vi "HFRR ADV v036.vi"() -> ()   [LabVIEW 2025] (continued)
                n905 = Match Pattern(string=w1143, regular expression=" \"width_px\":") -> (after substring=w1141:string)  [unwired: 1 in, 3 out]
                n906 = Match Pattern(string=w1141, regular expression="\"height_px\":") -> (before substring=w1139:string, after substring=w1138:string)  [unwired: 1 in, 2 out]
                n907 = Fract/Exp String To Number(string=w1139, default (0 dbl)=w1137) -> (number=w1136:dbl)  [unwired: 2 in, 1 out]
                n908 = Fract/Exp String To Number(string=w1138, default (0 dbl)=w1137) -> (number=w1135:dbl)  [unwired: 2 in, 1 out]
                n909 = Multiply(x=w1136, y=w1134) -> (x*y=w1133:dbl)
                n910 = Multiply(x=w1135, y=w1134) -> (x*y=w1132:dbl)
                n911 = Multiply(x=w1133, y=w1131) -> (x*y=w1117:dbl)
                n912 = Multiply(x=w1132, y=w1131) -> (x*y=w1115:dbl)
                n913 = Add(x=w1117, y=w1115) -> (x+y=w1129:dbl)
                n914 = property on="Major Axis" class="DigNum (strict)"("Caption.Text"="Major Axis") -> ()  [unwired: 2 in, 2 out]
                n915 = property on="Minor Axis" class="DigNum (strict)"("Caption.Text"="Minor Axis") -> ()  [unwired: 2 in, 2 out]
                n916 = property on="Average" class="DigNum (strict)"("Caption.Text"="Average") -> ()  [unwired: 2 in, 2 out]
                n917 = Divide(x=w1129, y=2.0) -> (x/y=w1113:dbl)
                n918 = Bundle By Name(cluster=w1130, "major"=w1117, "minor"=w1115, "average"=w1113) -> (w1127:cluster{"major":dbl, "minor":dbl, "average":dbl})
                n919 = Number To Fractional String(number=w1115, precision (6)=i16 1) -> (F-format string=w1122:string)  [unwired: 2 in]
                n920 = Number To Fractional String(number=w1113, precision (6)=i16 1) -> (F-format string=w1123:string)  [unwired: 2 in]
                n921 = Number To Fractional String(number=w1117, precision (6)=i16 1) -> (F-format string=w1121:string)  [unwired: 2 in]
                n922 = Fract/Exp String To Number(string=w1122) -> (number=w1114:dbl)  [unwired: 3 in, 1 out]
                n923 = Fract/Exp String To Number(string=w1123) -> (number=w1112:dbl)  [unwired: 3 in, 1 out]
                n924 = Fract/Exp String To Number(string=w1121) -> (number=w1116:dbl)  [unwired: 3 in, 1 out]
                n925 = local write "Major Axis"(w1116) -> ()
                n926 = local write "Average"(w1112) -> ()
                n927 = local write "Minor Axis"(w1114) -> ()
              }
            }
            n928 = case shown="\"Measrument\", Default" w1026 {
              tunnel: w1029 -> [w1056 _]
              tunnel: w1028 -> [w1055 _]
              tunnel: [w1052 w1081] -> w1027
              tunnel: w1025 -> [w1054 w1081]
              tunnel: w1024 -> [w1053 _]
              tunnel: w1021 -> [w1051 _]
              frame "Measrument", Default {
                n929 = stacked-sequence {
                  tunnel: w1056 -> [w1074 _]
                  tunnel: w1055 -> [w1072 _]
                  tunnel: w1054 -> [w1070 _]
                  tunnel: w1053 -> [w1069 _]
                  tunnel: [w1064 _] -> w1052
                  tunnel: w1051 -> [w1057 _]
                  frame #0 {
                    n930 = call "IMAGE ANALYSIS.vi"("Enum"=POST_ANALYSIS_ENUM."SAVE IMAGE", "error in"=w1070, "IMAGE FILE PATH"=w1069) -> ("error out"=w1068:errorcluster)  [unwired: 7 in, 1 out]
                    n931 = call "Stall Data Flow.vim"("value in"=w1068, "milliseconds to wait"=u32 1000) -> ("value out"=w1059:errorcluster)  [unwired: 1 out]
                    n932 = local read "Test File List :"() -> (w1076:string)
                    n933 = call "IMAGE ANALYSIS.vi"("Enum"=POST_ANALYSIS_ENUM."MINIMIZE UI", "error in"=w1059) -> ("error out"=w1066:errorcluster)  [unwired: 8 in, 1 out]
                    n934 = Bundle By Name(cluster=T27 {"File Name"="", "Test Method"="", "Operator"="", "Fuel Description"="", "Date and time"=""} ("Main Ref"), "Test Method"=w1057, "File Name"=w1076) -> (w1077:T27)
                    n935 = call "Stall Data Flow.vim"("value in"=w1066, "milliseconds to wait"=u32 1500) -> ("value out"=w1061:errorcluster)  [unwired: 1 out]
                    n936 = call "duf file read.vi"("error in (no error)"=w1061, "Main Ref"=w1077) -> ("error out"=w1075:errorcluster, "Main Ref 2"=w1073:T27)  [unwired: 8 in]
                    n937 = call "DETECTION REPORT for manual.vi"("error in (no error)"=w1075, "return value 3"=w1072, "Image File Path"=w1074, "Main Ref"=w1073) -> ("error out"=w1071:errorcluster)  [unwired: 7 in]
                    n938 = call <vilib>:"Clear Errors.vi"("error in (no error)"=w1071) -> ("error out"=w1062:errorcluster)  [unwired: 5 in, 1 out]
                    n939 = call "IMAGE ANALYSIS.vi"("Enum"=POST_ANALYSIS_ENUM."MINIMIZE UI", "error in"=w1062) -> ("error out"=w1064:errorcluster)  [unwired: 8 in, 1 out]
                  }
                  frame #1 {
                    n940 = local write "Main Tab"(T2."HOME" ("Main Tab")) -> ()
                    n941 = local write "Main Dashboard Buttons"(T1."Home" ("Main Dashboard Buttons")) -> ()
                  }
                }
              }
              frame "Calibrate" {
              }
            }
          }
          frame #2 {
            n942 = Not(x=w1146) -> (.not. x?=w1145:bool)
            n943 = local write "Confirm Measrurement"(w1145) -> ()
            n944 = local read "Calibration Tab"() -> (w1144:enum32{"Measrument", "Calibrate"})
            n945 = case shown="\"Measrument\", Default" w1144 {
              frame "Measrument", Default {
                (unwired) T21."HOME" ("Main Tab")
                n946 = local write "Main Tab"(T2."HOME" ("Main Tab")) -> ()
              }
              frame "Calibrate" {
              }
            }
          }
        }
      }
    }
    n947 = local read "Humidity"() -> (w889:bool)
    n948 = local read "Save Change"() -> (w894:bool)
    n949 = local read "Calibrate"() -> (w895:bool)
    n950 = local read "Auto Start Test"() -> (w890:bool)
    n951 = case shown="True" w895 {
      selector: w895 -> [_ w1002]
      frame False {
      }
      frame True {
        n952 = Not(x=w1002) -> (.not. x?=w1001:bool)
        n953 = local write "Calibrate"(w1001) -> ()
        n954 = local write "Calibration Tab"(enum32{"Measrument", "Calibrate"}."Calibrate" ("Calibration Tab")) -> ()
      }
    }
    n955 = case shown="True" w894 {
      selector: w894 -> [_ w946]
      frame False {
      }
      frame True {
        n956 = stacked-sequence {
          tunnel: w946 -> [_ _ _ _ w1000]
          frame #0 {
            n957 = call "IMAGE ANALYSIS.vi"("Enum"=POST_ANALYSIS_ENUM."HIDE UI") -> ()  [unwired: 9 in, 2 out]
          }
          frame #1 {
            n958 = local read "100x gain"() -> (w948:dbl)
            n959 = local read "10x Gain"() -> (w949:dbl)
            n960 = local read "5x Gain"() -> (w950:dbl)
            n961 = Number To Fractional String(number=w949, width (-)=i16 4, precision (6)=i16 7) -> (F-format string=w971:string)  [unwired: 1 in]
            n962 = Number To Fractional String(number=0.0, width (-)=i16 4, precision (6)=i16 7) -> (F-format string=w966:string)  [unwired: 1 in]
            n963 = Number To Fractional String(number=w948, width (-)=i16 4, precision (6)=i16 7) -> (F-format string=w954:string)  [unwired: 1 in]
            n964 = Number To Fractional String(number=w950, width (-)=i16 10 ("precision (6)"), precision (6)=i16 7) -> (F-format string=w980:string)  [unwired: 1 in]
            n965 = Concatenate Strings("[CH1]" ("string"), w980, " - 5x Gain" ("string"), "\r") -> (w970:string)
            n966 = Concatenate Strings("[CH2]" ("string"), w971, " - 10x Gain" ("string"), "\r") -> (w969:string)
            n967 = Concatenate Strings("[CH3]" ("string"), w966, " - 20x Gain" ("string"), "\r") -> (w960:string)
            n968 = Concatenate Strings("[CH4]" ("string"), w954, " - 100x Gain" ("string"), "\r") -> (w953:string)
            n969 = String To Path(string="C:\\LAB-IQ\\Image Calibrate v01.dcf") -> (path=w983:path)
            n970 = Concatenate Strings(w970, w969, w960, w953) -> (w968:string)
            n971 = call <vilib>:"Write Characters To File.vi"("append to file? (new file:F)"=FALSE, "character string"=w968, "file path (dialog if empty)"=w983) -> ()  [unwired: 2 in, 1 out]
          }
          frame #2 {
            n972 = String To Path(string="C:\\LAB-IQ\\Image Calibrate v01.dcf") -> (path=w986:path)
            n973 = Open/Create/Replace File ("Open File")(file path (use dialog)=w986) -> (refnum out=w987:refnum<file>)  [unwired: 5 in, 2 out]
            n974 = for {
              N: 4 -> [_]
              tunnel: w987 -> [w993]
              i -> [w989]
              n975 = Read from Text File ("Read File")(file (use dialog)=w993) -> (text=w994:string)  [unwired: 3 in, 3 out]
              n976 = String Subset(string=w994, offset (0)=6, length (rest)=10 ("length (rest)")) -> (substring=w990:string)
              n977 = Fract/Exp String To Number(string=w990) -> (number=w988:dbl)  [unwired: 3 in, 1 out]
              n978 = case shown="3" w989 {
                tunnel: w988 -> [w995 w996 _ w997 _]
                frame 0 {
                  n979 = local write "5x Gain"(w995) -> ()
                }
                frame 1 {
                  n980 = local write "10x Gain"(w996) -> ()
                }
                frame 2 {
                }
                frame 3 {
                  n981 = local write "100x gain"(w997) -> ()
                }
                frame 4, Default {
                }
              }
            }
          }
          frame #3 {
            n982 = call "IMAGE ANALYSIS.vi"("Enum"=POST_ANALYSIS_ENUM."SHOW UI") -> ()  [unwired: 9 in, 2 out]
          }
          frame #4 {
            n983 = Not(x=w1000) -> (.not. x?=w999:bool)
            n984 = local write "Save Change"(w999) -> ()
          }
        }
      }
    }
    n985 = case shown="False" w890 {
      tunnel: w889 -> [w916 _]
      frame False {
        n986 = case shown="True" w916 {
          frame False {
          }
          frame True {
            n987 = local read "Set Humidity:"() -> (w920:dbl)
            n988 = local read "Set Humidity:"() -> (w923:dbl)
            n989 = local read "Humidity ( %RH )"() -> (w924:dbl)
            n990 = Subtract(x=w920, y=2.0) -> (x-y=w918:dbl)
            n991 = Add(x=w923, y=2.0) -> (x+y=w919:dbl)
            n992 = In Range and Coerce(upper limit=w919, x=w924, lower limit=w918) -> (In Range?=w917:bool)  [unwired: 1 out]
            n993 = case shown="True" w917 {
              frame False {
              }
              frame True {
                n994 = case shown="True" "Manual Humididty Reached" {
                  selector: "Manual Humididty Reached" -> [_ w927]
                  frame False {
                  }
                  frame True {
                    n995 = Not(x=w927) -> (.not. x?=w926:bool)
                    n996 = local write "Manual Humididty Reached"(w926) -> ()
                    n997 = local read "EVENT LOG"() -> (w929:string)
                    n998 = call "Event Log.vi"("Content"="Target Humidity reached", "EVENT LOG"=w929) -> ("EVENT LOG"=w928:string)  [unwired: 8 in, 1 out]
                    n999 = local write "EVENT LOG"(w928) -> ()
                  }
                }
              }
            }
          }
        }
      }
      frame True {
        n1000 = local write "Manual Humididty Reached"(TRUE ("Manual Humididty Reached")) -> ()
      }
    }
    n1001 = local read "Cap Live Image"() -> (w910:bool)
    n1002 = local read "SCAR MEASURMENT"() -> (w913:enum32{"Auto Scar", "Manual Scar"})
    n1003 = Wait (ms)(milliseconds to wait=u32 250) -> ()  [unwired: 1 out]
    n1004 = Equal?(x=w913, y=enum32{"Auto Scar", "Manual Scar"}."Manual Scar" ("SCAR MEASURMENT")) -> (x = y?=w911:bool)
    n1005 = And(x=w911, y=w910) -> (x .and. y?=w909:bool)
    n1006 = case shown="True" w909 {
      selector: w909 -> [_ w1225]
      frame False {
      }
      frame True {
        n1007 = stacked-sequence {
          tunnel: [_ _ _ w1240 _] -> _
          tunnel: w1225 -> [_ _ _ _ w1247]
          frame #0 {
            w1226 = 0.0
            n1008 = local write "Major Axis"(w1226) -> ()
            n1009 = local write "Minor Axis"(w1226) -> ()
            n1010 = local write "Average"(w1226) -> ()
          }
          frame #1 {
            n1011 = call "CAMERA LIVE FEED FGV.vi"("Enum - Menu"=CAMERA_LIVE_FEED_ENUM."CAMERA MINIMIZE") -> ()  [unwired: 9 in, 2 out]
          }
          frame #2 {
            n1012 = local read "FILE 3"() -> (w1234:string)
            n1013 = call <vilib>:"Trim Whitespace.vi"("string"="C:\\LAB-IQ\\images\\") -> ("trimmed string"=w1236:string)  [unwired: 1 in]
            n1014 = String To Path(string=w1236) -> (path=w1235:path)
            n1015 = Concatenate Strings(w1234, ".png" ("string")) -> (w1233:string)
            n1016 = Build Path(base path=w1235, name or relative path=w1233) -> (appended path=w1231:path)
            n1017 = Path To String(path=w1231) -> (string=w1230:string)
            n1018 = call "CAMERA LIVE FEED FGV.vi"("Enum - Menu"=CAMERA_LIVE_FEED_ENUM."CAMERA SAVE", "Image Path"=w1230) -> ("error out"=w1228:errorcluster)  [unwired: 8 in, 1 out]
            n1019 = case shown="No Error" w1228 {
              frame No Error {
                n1020 = One Button Dialog(message="Image saved successfully") -> ()  [unwired: 1 in, 1 out]
              }
              frame Error {
              }
            }
          }
          frame #3 {
            n1021 = call "LIST FILE NAMES.vi"() -> ("error out"=w1242:errorcluster, "filenames"=w1239:string[])  [unwired: 10 in]
            n1022 = call "IMAGE ANALYSIS.vi"("Enum"=POST_ANALYSIS_ENUM."SHOW UI", "error in"=w1242) -> ("error out"=w1240:errorcluster)  [unwired: 8 in, 1 out]
            n1023 = property on="Test File List :" class="CmbBox"("Strings[]"=w1239) -> ()  [unwired: 2 in, 2 out]
          }
          frame #4 {
            (unwired) T26."Report" ("Main Dashboard Buttons")
            (unwired) T28."Report" ("Main Dashboard Buttons")
            n1024 = Not(x=w1247) -> (.not. x?=w1246:bool)
            n1025 = local write "Zoom Factore"(0.0 ("Zoom Factore")) -> ()
            n1026 = local write "Cap Live Image"(w1246) -> ()
            n1027 = local write "Main Tab"(T2."Adv Scar Report" ("Main Tab")) -> ()
            n1028 = property on="Cap Live Image" class="Bool (strict)"("BoolText.Text"="Capture Image" ("Boolean Text.Text")) -> ()  [unwired: 2 in, 2 out]
            n1029 = local write "Main Dashboard Buttons"(T1."Report" ("Main Dashboard Buttons")) -> ()
          }
        }
      }
    }
    n1030 = local read "change Gain"() -> (w893:bool)
    n1031 = local read "Back Square"() -> (w892:bool)
    n1032 = case shown="True" w893 {
      selector: w893 -> [_ w937]
      frame False {
      }
      frame True {
        n1033 = stacked-sequence {
          tunnel: w937 -> [_ w945]
          frame #0 {
            n1034 = local read "Actual (µm)"() -> (w941:dbl)
            n1035 = local read "Pixel Value"() -> (w940:dbl)
            n1036 = local read "Magnification :"() -> (w939:string)
            n1037 = Divide(x=w941, y=w940) -> (x/y=w938:dbl)
            n1038 = case shown="\"10x\"" w939 {
              tunnel: w938 -> [w942 w943]
              frame "10x" {
                n1039 = local write "10x Gain"(w942) -> ()
              }
              frame "5x", Default {
                n1040 = local write "5x Gain"(w943) -> ()
              }
            }
          }
          frame #1 {
            n1041 = Not(x=w945) -> (.not. x?=w944:bool)
            n1042 = local write "change Gain"(w944) -> ()
          }
        }
      }
    }
    n1043 = case shown="True" w892 {
      selector: w892 -> [_ w935]
      frame False {
      }
      frame True {
        n1044 = Not(x=w935) -> (.not. x?=w934:bool)
        n1045 = local write "Back Square"(w934) -> ()
        n1046 = local write "Calibration Tab"(enum32{"Measrument", "Calibrate"}."Measrument" ("Calibration Tab")) -> ()
      }
    }
    n1047 = local read "Rectangle Tool"() -> (w904:bool)
    n1048 = local read "Clear ROI Tool"() -> (w903:bool)
    n1049 = local read "Open Image"() -> (w908:bool)
    n1050 = local read "line tool"() -> (w905:bool)
    n1051 = local read "OUT"() -> (w906:bool)
    n1052 = local read "In"() -> (w907:bool)
    n1053 = case shown="True" w908 {
      selector: w908 -> [_ w1213]
      tunnel: [w1209 w1215] -> _
      tunnel: w898 -> [w1209 w1214]
      frame False {
      }
      frame True {
        n1054 = Not(x=w1213) -> (.not. x?=w1212:bool)
        n1055 = local write "Open Image"(w1212) -> ()
        n1056 = call "IMAGE ANALYSIS.vi"("Enum"=POST_ANALYSIS_ENUM."HIDE UI", "error in"=w1214) -> ("error out"=w1222:errorcluster)  [unwired: 8 in, 1 out]
        n1057 = call "File Dialog"("start path"=path "C:/LAB-IQ/images", "error in"=w1222) -> ("selected path"=w1211:path, "error out"=w1220:errorcluster)  [unwired: 10 in, 2 out]
        "Image path  2" <- w1211
        n1058 = call <vilib>:"Clear Errors.vi"("error in (no error)"=w1220) -> ("error out"=w1219:errorcluster)  [unwired: 5 in, 1 out]
        n1059 = call "IMAGE ANALYSIS.vi"("Enum"=POST_ANALYSIS_ENUM."OPEN FILE", "error in"=w1219, "File Path"=w1211) -> ("error out"=w1218:errorcluster)  [unwired: 7 in, 1 out]
        n1060 = call <vilib>:"Clear Errors.vi"("error in (no error)"=w1218) -> ("error out"=w1217:errorcluster)  [unwired: 5 in, 1 out]
        n1061 = call "IMAGE ANALYSIS.vi"("Enum"=POST_ANALYSIS_ENUM."SHOW UI", "error in"=w1217) -> ("error out"=w1215:errorcluster)  [unwired: 8 in, 1 out]
        n1062 = local write "Zoom Factore"(100.0 ("Zoom Factore")) -> ()
      }
    }
    n1063 = case shown="True" w906 {
      selector: w906 -> [_ w1194]
      tunnel: w898 -> [w1191 w1199]
      tunnel: [w1191 w1193] -> _
      frame False {
      }
      frame True {
        n1064 = Not(x=w1194) -> (.not. x?=w1192:bool)
        n1065 = local read "Zoom Factore"() -> (w1197:dbl)
        n1066 = local write "OUT"(w1192) -> ()
        n1067 = call "IMAGE ANALYSIS.vi"("Enum"=POST_ANALYSIS_ENUM."ZOOM OUT", "error in"=w1199) -> ("error out"=w1193:errorcluster)  [unwired: 8 in, 1 out]
        n1068 = Divide(x=w1197, y=1.2) -> (x/y=w1195:dbl)
        n1069 = local write "Zoom Factore"(w1195) -> ()
      }
    }
    n1070 = case shown="True" w907 {
      selector: w907 -> [_ w1203]
      tunnel: w898 -> [w1200 w1208]
      tunnel: [w1200 w1201] -> _
      frame False {
      }
      frame True {
        n1071 = Not(x=w1203) -> (.not. x?=w1202:bool)
        n1072 = local read "Zoom Factore"() -> (w1206:dbl)
        n1073 = local write "In"(w1202) -> ()
        n1074 = call "IMAGE ANALYSIS.vi"("Enum"=POST_ANALYSIS_ENUM."ZOOM IN", "error in"=w1208) -> ("error out"=w1201:errorcluster)  [unwired: 8 in, 1 out]
        n1075 = Multiply(x=w1206, y=1.2) -> (x*y=w1204:dbl)
        n1076 = local write "Zoom Factore"(w1204) -> ()
      }
    }
    n1077 = case shown="True" w903 {
      selector: w903 -> [_ w1175]
      tunnel: w898 -> [w1173 w1177]
      tunnel: [w1173 w1176] -> _
      frame False {
      }
      frame True {
        n1078 = Not(x=w1175) -> (.not. x?=w1174:bool)
        n1079 = local write "Clear ROI Tool"(w1174) -> ()
        n1080 = call "IMAGE ANALYSIS.vi"("Enum"=POST_ANALYSIS_ENUM."CLEAR ROI", "error in"=w1177) -> ("error out"=w1176:errorcluster)  [unwired: 8 in, 1 out]
      }
    }
    n1081 = case shown="True" w905 {
      selector: w905 -> [_ w1187]
      tunnel: w898 -> [w1185 w1190]
      tunnel: [w1185 w1188] -> _
      frame False {
      }
      frame True {
        n1082 = Not(x=w1187) -> (.not. x?=w1186:bool)
        n1083 = local write "line tool"(w1186) -> ()
        n1084 = call "IMAGE ANALYSIS.vi"("Enum"=POST_ANALYSIS_ENUM."DRAW LINE", "error in"=w1190) -> ("error out"=w1188:errorcluster)  [unwired: 8 in, 1 out]
      }
    }
    n1085 = case shown="True" w904 {
      selector: w904 -> [_ w1181]
      tunnel: w898 -> [w1179 w1183]
      tunnel: [w1179 w1182] -> _
      frame False {
      }
      frame True {
        n1086 = Not(x=w1181) -> (.not. x?=w1180:bool)
        n1087 = local write "Rectangle Tool"(w1180) -> ()
        n1088 = call "IMAGE ANALYSIS.vi"("Enum"=POST_ANALYSIS_ENUM."DRAW REC", "error in"=w1183) -> ("error out"=w1182:errorcluster)  [unwired: 8 in, 1 out]
      }
    }
    n1089 = local read "SCAR MEASURMENT"() -> (w891:enum32{"Auto Scar", "Manual Scar"})
    n1090 = local read "Fit to Screen Tool"() -> (w900:bool)
    n1091 = local read "Resize Tool"() -> (w899:bool)
    n1092 = case shown="\"Manual Scar\", Default" w891 {
      frame "Auto Scar" {
        n1093 = property on="Cap Live Image" class="Bool (strict)"("BoolText.Text"="Report" ("Boolean Text.Text")) -> ()  [unwired: 2 in, 2 out]
      }
      frame "Manual Scar", Default {
        n1094 = property on="Cap Live Image" class="Bool (strict)"("BoolText.Text"="Save Image" ("Boolean Text.Text")) -> ()  [unwired: 2 in, 2 out]
      }
    }
    n1095 = local read "ROI Color Tool"() -> (w901:bool)
    n1096 = local read "Pan Tool"() -> (w902:bool)
    n1097 = case shown="True" w902 {
      selector: w902 -> [_ w1169]
      tunnel: w898 -> [w1167 w1171]
      tunnel: [w1167 w1170] -> _
      frame False {
      }
      frame True {
        n1098 = Not(x=w1169) -> (.not. x?=w1168:bool)
        n1099 = call "IMAGE ANALYSIS.vi"("Enum"=POST_ANALYSIS_ENUM."PAN", "error in"=w1171) -> ("error out"=w1170:errorcluster)  [unwired: 8 in, 1 out]
        n1100 = local write "Pan Tool"(w1168) -> ()
      }
    }
    n1101 = case shown="True" w899 {
      selector: w899 -> [_ w1153]
      tunnel: w898 -> [w1148 w1150]
      tunnel: [w1148 w1149] -> _
      frame False {
      }
      frame True {
        n1102 = Not(x=w1153) -> (.not. x?=w1152:bool)
        n1103 = local write "Resize Tool"(w1152) -> ()
        n1104 = call "IMAGE ANALYSIS.vi"("Enum"=POST_ANALYSIS_ENUM."RESIZE MODE", "error in"=w1150) -> ("error out"=w1149:errorcluster)  [unwired: 8 in, 1 out]
      }
    }
    n1105 = case shown="True" w900 {
      selector: w900 -> [_ w1158]
      tunnel: [w1154 w1159] -> _
      tunnel: w898 -> [w1154 w1157]
      frame False {
      }
      frame True {
        n1106 = Not(x=w1158) -> (.not. x?=w1156:bool)
        n1107 = local write "Zoom Factore"(100.0 ("Zoom Factore")) -> ()
        n1108 = local write "Fit to Screen Tool"(w1156) -> ()
        n1109 = call "IMAGE ANALYSIS.vi"("Enum"=POST_ANALYSIS_ENUM."FIT", "error in"=w1157) -> ("error out"=w1159:errorcluster)  [unwired: 8 in, 1 out]
      }
    }
    n1110 = case shown="True" w901 {
      selector: w901 -> [_ w1164]
      tunnel: [w1161 w1165] -> _
      tunnel: w898 -> [w1161 w1162]
      frame False {
      }
      frame True {
        n1111 = Not(x=w1164) -> (.not. x?=w1163:bool)
        n1112 = local write "ROI Color Tool"(w1163) -> ()
        n1113 = call "IMAGE ANALYSIS.vi"("Enum"=POST_ANALYSIS_ENUM."SET ROI COLOR", "error in"=w1162) -> ("error out"=w1165:errorcluster)  [unwired: 8 in, 1 out]
      }
    }
    n1114 = local read "Quit"() -> (w915:bool)
  }
  n1115 = while {
    stop <- w1249 stop-if-true
    n1116 = local read "Image Path"() -> (w1252:path)
    n1117 = local read "Print 3"() -> (w1255:bool)
    n1118 = Equal?(x=w1252, y=path "") -> (x = y?=w1251:bool)
    n1119 = Not(x=w1251) -> (.not. x?=w1250:bool)
    n1120 = property on="Print 3" class="Bool (strict)"("Visible"=w1250) -> ()  [unwired: 2 in, 2 out]
    n1121 = case shown="True" w1255 {
      frame False {
        n1122 = local write "Rd"(TRUE ("Boolean 7")) -> ()
      }
      frame True {
        n1123 = flat-sequence {
          tunnel: [w1295] -> w1263
          tunnel: [w1282] -> w1261
          tunnel: [w1292] -> w1257
          tunnel: w1263 -> [w1304]
          tunnel: [w1304] -> w1262
          tunnel: w1261 -> [w1303]
          tunnel: [w1303] -> w1260
          tunnel: [w1301] -> w1259
          tunnel: [w1300] -> w1258
          tunnel: w1257 -> [w1300]
          tunnel: w1262 -> [w1306]
          tunnel: w1260 -> [w1307]
          tunnel: w1259 -> [_]
          tunnel: w1258 -> [w1305]
          frame #0 {
            n1124 = case shown="True" "Rd" {
              frame False {
              }
              frame True {
                n1125 = while {
                  tunnel: "abcdefABCDEF" ("string 2") -> [w1274]
                  shift-right: [w1272] -> w1266
                  shift-left: "" -> [w1271]
                  i -> [w1281]
                  stop <- w1280 stop-if-true
                  n1126 = Random Number (0-1)() -> (number: 0 to 1=w1275:dbl)
                  n1127 = Multiply(x=w1275, y=62.0) -> (x*y=w1277:dbl)
                  n1128 = Decrement(x="Length 2") -> (x-1=w1270:i16)
                  n1129 = To Word Integer(number=w1277) -> (16bit integer=w1278:i16)
                  n1130 = String Subset(string=w1274, offset (0)=w1278, length (rest)=1 ("length (rest)")) -> (substring=w1273:string)
                  n1131 = Greater Or Equal?(x=w1281, y=w1270) -> (x >= y?=w1280:bool)
                  n1132 = Concatenate Strings(w1273, w1271) -> (w1272:string)
                }
                "String 10" <- w1266
                n1133 = local write "Rd"(FALSE ("Boolean 7")) -> ()
              }
            }
          }
          frame #1 {
            w1293 = "_resized.jpg" ("command line")
            (unwired) ".jpg -resize 320x240 " ("string")
            (unwired) "Choose an Image File" ("prompt")
            # "-resize 1798x425"
            n1134 = local read "Image Path"() -> (w1287:path)
            n1135 = Strip Path(path=w1287) -> (stripped path=w1282:path, name=w1283:string)
            n1136 = Match Pattern(string=w1283, regular expression=".jpg") -> (before substring=→"before substring 2":string, after substring=→"after substring":string)  [unwired: 1 in, 2 out]
            n1137 = Match Pattern(string=w1283, regular expression="\\") -> (before substring=w1289:string)  [unwired: 1 in, 3 out]
            n1138 = Match Pattern(string=w1289, regular expression=".jpg") -> (before substring=w1288:string)  [unwired: 1 in, 3 out]
            n1139 = Concatenate Strings("cmd /c convert " ("string"), w1288, ".jpg -resize 320x240  " ("command line"), w1288, w1293) -> (w1296:string)
            n1140 = call <vilib>:"System Exec.vi"("run minimized? (F)"=TRUE, "wait until completion? (T)"=TRUE, "working directory"=w1282, "command line"=w1296) -> ("error out"=w1295:errorcluster)  [unwired: 4 in, 3 out]
            "error out 2" <- w1295
            n1141 = Concatenate Strings(w1288, w1293) -> (w1292:string)
          }
          frame #2 {
            n1142 = Wait (ms)(milliseconds to wait=u32 2000 ("millisecond timer value")) -> (millisecond timer value=w1301:u32)
          }
          frame #3 {
            n1143 = case shown="No Error" w1306 {
              tunnel: w1307 -> [w1310 _]
              tunnel: w1305 -> [w1308 _]
              frame No Error {
                (unwired) ".jpg" ("string")
                n1144 = Path To String(path=w1310) -> (string=w1314:string)
                n1145 = Concatenate Strings(w1314, "\\" ("string"), w1308) -> (w1313:string)
                n1146 = String To Path(string=w1313) -> (path=w1312:path)
                n1147 = call <vilib>:"Read JPEG File.vi"("path to JPEG file"=w1312) -> ("image data"=w1316:T16)  [unwired: 8 in, 2 out]
                "image data" <- w1316
                n1148 = local write "Print 3"(FALSE ("Print 2")) -> ()
                n1149 = call <vilib>:"Draw Flattened Pixmap.vi"("image data"=w1316) -> ("new picture"=→"new picture":picture)  [unwired: 8 in]
              }
              frame Error {
              }
            }
          }
        }
      }
    }
    n1150 = Wait (ms)(milliseconds to wait=u32 20 ("millisecond timer value")) -> ()  [unwired: 1 out]
    n1151 = local read "Quit"() -> (w1249:bool)
  }
  n1152 = while {
    tunnel: w38 -> [_]
    tunnel: w24 -> [_]
    stop <- w1346 stop-if-true
    # "New Adv Logics"
    n1153 = local read "Main Tab"() -> (w1327:T2)
    n1154 = local read "Main Tab"() -> (w1344:T2)
    n1155 = local read "Sign In"() -> (w1343:bool)
    n1156 = case shown="\"Adv Scar\"" w1327 {
      frame "HOME", Default {
        n1157 = local read "LIVE FEED MIN TEMP"() -> (w1479:bool)
        n1158 = local write "LIVE FEED MAX TEMP"(TRUE ("LIVE FEED MAX TEMP")) -> ()
        n1159 = local read "CAMERA ROI MIN TEMP"() -> (w1477:bool)
        n1160 = case shown="True" w1479 {
          selector: w1479 -> [_ w1486]
          frame False {
          }
          frame True {
            n1161 = Not(x=w1486) -> (.not. x?=w1485:bool)
            n1162 = local write "LIVE FEED MIN TEMP"(w1485) -> ()
            n1163 = call "CAMERA LIVE FEED FGV.vi"("Enum - Menu"=CAMERA_LIVE_FEED_ENUM."CAMERA MINIMIZE") -> ()  [unwired: 9 in, 2 out]
          }
        }
        n1164 = case shown="True" w1477 {
          selector: w1477 -> [_ w1483]
          frame False {
          }
          frame True {
            n1165 = Not(x=w1483) -> (.not. x?=w1482:bool)
            n1166 = local write "CAMERA ROI MIN TEMP"(w1482) -> ()
            n1167 = call "IMAGE ANALYSIS.vi"("Enum"=POST_ANALYSIS_ENUM."MINIMIZE UI") -> ()  [unwired: 9 in, 2 out]
          }
        }
        n1168 = local write "CAMERA ROI MAX TEMP"(TRUE ("CAMERA ROI MAX TEMP")) -> ()
      }
      frame "Test Setup" {
        n1169 = local read "LIVE FEED MIN TEMP"() -> (w1489:bool)
        n1170 = local read "CAMERA ROI MIN TEMP"() -> (w1487:bool)
        n1171 = local write "LIVE FEED MAX TEMP"(TRUE ("LIVE FEED MAX TEMP")) -> ()
        n1172 = case shown="True" w1489 {
          selector: w1489 -> [_ w1496]
          frame False {
          }
          frame True {
            n1173 = Not(x=w1496) -> (.not. x?=w1495:bool)
            n1174 = local write "LIVE FEED MIN TEMP"(w1495) -> ()
            n1175 = call "CAMERA LIVE FEED FGV.vi"("Enum - Menu"=CAMERA_LIVE_FEED_ENUM."CAMERA MINIMIZE") -> ()  [unwired: 9 in, 2 out]
          }
        }
        n1176 = case shown="True" w1487 {
          selector: w1487 -> [_ w1493]
          frame False {
          }
          frame True {
            n1177 = Not(x=w1493) -> (.not. x?=w1492:bool)
            n1178 = local write "CAMERA ROI MIN TEMP"(w1492) -> ()
            n1179 = call "IMAGE ANALYSIS.vi"("Enum"=POST_ANALYSIS_ENUM."MINIMIZE UI") -> ()  [unwired: 9 in, 2 out]
          }
        }
        n1180 = local write "CAMERA ROI MAX TEMP"(TRUE ("CAMERA ROI MAX TEMP")) -> ()
      }
      frame "Acquire" {
        n1181 = local read "LIVE FEED MIN TEMP"() -> (w1499:bool)
        n1182 = local write "LIVE FEED MAX TEMP"(TRUE ("LIVE FEED MAX TEMP")) -> ()
        n1183 = local read "CAMERA ROI MIN TEMP"() -> (w1497:bool)
        n1184 = case shown="True" w1499 {
          selector: w1499 -> [_ w1506]
          frame False {
          }
          frame True {
            n1185 = Not(x=w1506) -> (.not. x?=w1505:bool)
            n1186 = local write "LIVE FEED MIN TEMP"(w1505) -> ()
            n1187 = call "CAMERA LIVE FEED FGV.vi"("Enum - Menu"=CAMERA_LIVE_FEED_ENUM."CAMERA MINIMIZE") -> ()  [unwired: 9 in, 2 out]
          }
        }
        n1188 = case shown="True" w1497 {
          selector: w1497 -> [_ w1503]
          frame False {
          }
          frame True {
            n1189 = Not(x=w1503) -> (.not. x?=w1502:bool)
            n1190 = local write "CAMERA ROI MIN TEMP"(w1502) -> ()
            n1191 = call "IMAGE ANALYSIS.vi"("Enum"=POST_ANALYSIS_ENUM."MINIMIZE UI") -> ()  [unwired: 9 in, 2 out]
          }
        }
        n1192 = local write "CAMERA ROI MAX TEMP"(TRUE ("CAMERA ROI MAX TEMP")) -> ()
      }
      frame "Adv Scar" {
        n1193 = local read "CAMERA ROI MIN TEMP"() -> (w1507:bool)
        n1194 = case shown="True" "LIVE FEED MAX TEMP" {
          selector: "LIVE FEED MAX TEMP" -> [_ w1528]
          frame False {
          }
          frame True {
            n1195 = Not(x=w1528) -> (.not. x?=w1527:bool)
            n1196 = local write "LIVE FEED MAX TEMP"(w1527) -> ()
            n1197 = call "CAMERA LIVE FEED FGV.vi"("Enum - Menu"=CAMERA_LIVE_FEED_ENUM."CAMERA RESTORE") -> ("error out"=w1518:errorcluster)  [unwired: 9 in, 1 out]
            n1198 = Type Cast(type=30, x=0) -> (*(type *) &x=w1522:i32)
            n1199 = Add(x=w1522, y=48) -> (x+y=w1523:i32)
            n1200 = call "CAMERA LIVE FEED FGV.vi"("Enum - Menu"=CAMERA_LIVE_FEED_ENUM."CAMERA MODE SET", "error in (no error)"=w1518, "CAMERA MODE"=w1523) -> ("error out"=w1515:errorcluster)  [unwired: 7 in, 1 out]
            n1201 = call "CAMERA LIVE FEED FGV.vi"("Enum - Menu"=CAMERA_LIVE_FEED_ENUM."CAMERA GRAY", "error in (no error)"=w1515) -> ("error out"=w1514:errorcluster)  [unwired: 8 in, 1 out]
            n1202 = call "LIST FILE NAMES.vi"("error in (no error)"=w1514) -> ("error out"=w1524:errorcluster, "filenames"=w1525:string[])  [unwired: 9 in]
            n1203 = property on="FILE 3" class="CmbBox"(error in=w1524, "Strings[]"=w1525) -> ()  [unwired: 1 in, 2 out]
          }
        }
        n1204 = case shown="True" w1507 {
          selector: w1507 -> [_ w1513]
          frame False {
          }
          frame True {
            n1205 = Not(x=w1513) -> (.not. x?=w1512:bool)
            n1206 = local write "CAMERA ROI MIN TEMP"(w1512) -> ()
            n1207 = call "IMAGE ANALYSIS.vi"("Enum"=POST_ANALYSIS_ENUM."MINIMIZE UI") -> ()  [unwired: 9 in, 2 out]
          }
        }
        n1208 = local write "CAMERA ROI MAX TEMP"(TRUE ("CAMERA ROI MAX TEMP")) -> ()
        "LIVE FEED MIN TEMP" <- TRUE ("LIVE FEED MIN TEMP")
      }
      frame "Adv Scar Report" {
        n1209 = local read "CAMERA ROI MAX TEMP"() -> (w1529:bool)
        n1210 = local read "LIVE FEED MIN TEMP"() -> (w1531:bool)
        n1211 = local write "LIVE FEED MAX TEMP"(TRUE ("LIVE FEED MAX TEMP")) -> ()
        n1212 = case shown="True" w1531 {
          selector: w1531 -> [_ w1540]
          frame False {
          }
          frame True {
            n1213 = Not(x=w1540) -> (.not. x?=w1539:bool)
            n1214 = local write "LIVE FEED MIN TEMP"(w1539) -> ()
            n1215 = call "CAMERA LIVE FEED FGV.vi"("Enum - Menu"=CAMERA_LIVE_FEED_ENUM."CAMERA MINIMIZE") -> ()  [unwired: 9 in, 2 out]
          }
        }
        n1216 = case shown="True" w1529 {
          selector: w1529 -> [_ w1537]
          frame False {
          }
          frame True {
            n1217 = Not(x=w1537) -> (.not. x?=w1535:bool)
            n1218 = local write "CAMERA ROI MAX TEMP"(w1535) -> ()
            n1219 = call "IMAGE ANALYSIS.vi"("Enum"=POST_ANALYSIS_ENUM."SHOW UI") -> ("error out"=w1534:errorcluster)  [unwired: 9 in, 1 out]
            n1220 = call "LIST FILE NAMES.vi"("error in (no error)"=w1534) -> ("filenames"=w1533:string[])  [unwired: 9 in, 1 out]
            n1221 = property on="Test File List :" class="CmbBox"("Strings[]"=w1533) -> ()  [unwired: 2 in, 2 out]
          }
        }
        n1222 = local write "CAMERA ROI MIN TEMP"(TRUE ("CAMERA ROI MIN TEMP")) -> ()
      }
      frame "Compare Files" {
        n1223 = local read "LIVE FEED MIN TEMP"() -> (w1543:bool)
        n1224 = local write "LIVE FEED MAX TEMP"(TRUE ("LIVE FEED MAX TEMP")) -> ()
        n1225 = local read "CAMERA ROI MIN TEMP"() -> (w1541:bool)
        n1226 = case shown="True" w1543 {
          selector: w1543 -> [_ w1550]
          frame False {
          }
          frame True {
            n1227 = Not(x=w1550) -> (.not. x?=w1549:bool)
            n1228 = local write "LIVE FEED MIN TEMP"(w1549) -> ()
            n1229 = call "CAMERA LIVE FEED FGV.vi"("Enum - Menu"=CAMERA_LIVE_FEED_ENUM."CAMERA MINIMIZE") -> ()  [unwired: 9 in, 2 out]
          }
        }
        n1230 = case shown="True" w1541 {
          selector: w1541 -> [_ w1547]
          frame False {
          }
          frame True {
            n1231 = Not(x=w1547) -> (.not. x?=w1546:bool)
            n1232 = local write "CAMERA ROI MIN TEMP"(w1546) -> ()
            n1233 = call "IMAGE ANALYSIS.vi"("Enum"=POST_ANALYSIS_ENUM."MINIMIZE UI") -> ()  [unwired: 9 in, 2 out]
          }
        }
        n1234 = local write "CAMERA ROI MAX TEMP"(TRUE ("CAMERA ROI MAX TEMP")) -> ()
      }
      frame "About" {
        n1235 = local read "LIVE FEED MIN TEMP"() -> (w1553:bool)
        n1236 = local write "LIVE FEED MAX TEMP"(TRUE ("LIVE FEED MAX TEMP")) -> ()
        n1237 = local read "CAMERA ROI MIN TEMP"() -> (w1552:bool)
        n1238 = case shown="True" w1553 {
          selector: w1553 -> [_ w1560]
          frame False {
          }
          frame True {
            n1239 = Not(x=w1560) -> (.not. x?=w1559:bool)
            n1240 = local write "LIVE FEED MIN TEMP"(w1559) -> ()
            n1241 = call "CAMERA LIVE FEED FGV.vi"("Enum - Menu"=CAMERA_LIVE_FEED_ENUM."CAMERA MINIMIZE") -> ()  [unwired: 9 in, 2 out]
          }
        }
        n1242 = case shown="True" w1552 {
          selector: w1552 -> [_ w1557]
          frame False {
          }
          frame True {
            n1243 = Not(x=w1557) -> (.not. x?=w1556:bool)
            n1244 = local write "CAMERA ROI MIN TEMP"(w1556) -> ()
            n1245 = call "IMAGE ANALYSIS.vi"("Enum"=POST_ANALYSIS_ENUM."MINIMIZE UI") -> ()  [unwired: 9 in, 2 out]
          }
        }
        n1246 = local write "CAMERA ROI MAX TEMP"(TRUE ("CAMERA ROI MIN TEMP")) -> ()
      }
      frame "Advance" {
        n1247 = local read "LIVE FEED MIN TEMP"() -> (w1563:bool)
        n1248 = local write "LIVE FEED MAX TEMP"(TRUE ("LIVE FEED MAX TEMP")) -> ()
        n1249 = local read "CAMERA ROI MIN TEMP"() -> (w1561:bool)
        n1250 = case shown="True" w1563 {
          selector: w1563 -> [_ w1570]
          frame False {
          }
          frame True {
            n1251 = Not(x=w1570) -> (.not. x?=w1569:bool)
            n1252 = local write "LIVE FEED MIN TEMP"(w1569) -> ()
            n1253 = call "CAMERA LIVE FEED FGV.vi"("Enum - Menu"=CAMERA_LIVE_FEED_ENUM."CAMERA MINIMIZE") -> ()  [unwired: 9 in, 2 out]
          }
        }
        n1254 = local write "CAMERA ROI MAX TEMP"(TRUE ("CAMERA ROI MAX TEMP")) -> ()
        n1255 = case shown="True" w1561 {
          selector: w1561 -> [_ w1567]
          frame False {
          }
          frame True {
            n1256 = Not(x=w1567) -> (.not. x?=w1566:bool)
            n1257 = local write "CAMERA ROI MIN TEMP"(w1566) -> ()
            n1258 = call "IMAGE ANALYSIS.vi"("Enum"=POST_ANALYSIS_ENUM."MINIMIZE UI") -> ()  [unwired: 9 in, 2 out]
          }
        }
      }
      frame "Mooha" {
        n1259 = local read "LIVE FEED MIN TEMP"() -> (w1573:bool)
        n1260 = local write "LIVE FEED MAX TEMP"(TRUE ("LIVE FEED MAX TEMP")) -> ()
        n1261 = local read "CAMERA ROI MIN TEMP"() -> (w1571:bool)
        n1262 = case shown="True" w1573 {
          selector: w1573 -> [_ w1580]
          frame False {
          }
          frame True {
            n1263 = Not(x=w1580) -> (.not. x?=w1579:bool)
            n1264 = local write "LIVE FEED MIN TEMP"(w1579) -> ()
            n1265 = call "CAMERA LIVE FEED FGV.vi"("Enum - Menu"=CAMERA_LIVE_FEED_ENUM."CAMERA MINIMIZE") -> ()  [unwired: 9 in, 2 out]
          }
        }
        n1266 = local write "CAMERA ROI MAX TEMP"(TRUE ("CAMERA ROI MAX TEMP")) -> ()
        n1267 = case shown="True" w1571 {
          selector: w1571 -> [_ w1577]
          frame False {
          }
          frame True {
            n1268 = Not(x=w1577) -> (.not. x?=w1576:bool)
            n1269 = local write "CAMERA ROI MIN TEMP"(w1576) -> ()
            n1270 = call "IMAGE ANALYSIS.vi"("Enum"=POST_ANALYSIS_ENUM."MINIMIZE UI") -> ()  [unwired: 9 in, 2 out]
          }
        }
      }
    }
    n1271 = local read "Auto Start Test"() -> (w1318:bool)
    n1272 = case shown="True" "sign in temp" {
      frame False {
      }
      frame True {
        w1353 = 1 ("y")
        n1273 = local read "USERNAME"() -> (w1359:string)
        n1274 = local read "USER ID"() -> (w1356:string)
        n1275 = call <vilib>:"Trim Whitespace.vi"("string"=w1359) -> ("trimmed string"=w1358:string)  [unwired: 1 in]
        n1276 = call <vilib>:"Trim Whitespace.vi"("string"=w1356) -> ("trimmed string"=w1357:string)  [unwired: 1 in]
        n1277 = String Length(string=w1358) -> (length=w1355:i32)
        n1278 = String Length(string=w1357) -> (length=w1354:i32)
        n1279 = Greater?(x=w1355, y=w1353) -> (0:w1352:bool)
        n1280 = Greater?(x=w1354, y=w1353) -> (0:w1351:bool)
        n1281 = And(x=w1352, y=w1351) -> (x .and. y?=w1350:bool)
        n1282 = case shown="True" w1350 {
          frame False {
            n1283 = property on="Sign In" class="Bool (strict)"("DisabledEnum"=T19."Disabled" ("Disabled")) -> ()  [unwired: 2 in, 2 out]
          }
          frame True {
            n1284 = property on="Sign In" class="Bool (strict)"("DisabledEnum"=T19."Enabled" ("Disabled")) -> ()  [unwired: 2 in, 2 out]
          }
        }
      }
    }
    n1285 = local read "Air Temperature"() -> (w1335:bool)
    n1286 = local read "Coefficient Of Friction"() -> (w1336:bool)
    n1287 = case shown="False" w1318 {
      frame False {
        n1288 = local read "Auto stop temp"() -> (w1347:bool)
        n1289 = case shown="True" w1347 {
          frame False {
          }
          frame True {
            n1290 = local write "Auto Start Temp"(FALSE ("Auto Start Temp")) -> ()
          }
        }
      }
      frame True {
        "Auto stop temp" <- TRUE ("Auto stop temp")
      }
    }
    n1291 = local read "Humidity"() -> (w1334:bool)
    n1292 = case shown="\"HOME\"" w1344 {
      frame "HOME" {
        n1293 = local write "main tab sub"(enum32{"Page 1", "Page 2"}."Page 1" ("main tab sub")) -> ()
      }
      frame Default {
        n1294 = local write "main tab sub"(enum32{"Page 1", "Page 2"}."Page 2" ("main tab sub")) -> ()
      }
    }
    n1295 = case shown="True" w1343 {
      selector: w1343 -> [_ w1694]
      frame False {
      }
      frame True {
        n1296 = Not(x=w1694) -> (.not. x?=w1693:bool)
        n1297 = local write "Sign In"(w1693) -> ()
        n1298 = local write "Main Dashboard Buttons"(T26."Test Setup" ("Main Dashboard Buttons")) -> ()
      }
    }
    n1299 = case shown="\"Numeric Display\", Default" "Num/Graph" {
      frame "Numeric Display", Default {
        n1300 = property on="Single/Multiple" class="RadioBtnsControl (strict)"("Visible"=FALSE) -> ()  [unwired: 2 in, 2 out]
        n1301 = property on="Single - Graph" class="Ring (strict)"("Visible"=FALSE) -> ()  [unwired: 2 in, 2 out]
        n1302 = local write "Main Tab Display"(T4."Dashboard 1" ("Main Tab Display")) -> ()
      }
      frame "Graph Display" {
        n1303 = property on="Single/Multiple" class="RadioBtnsControl (strict)"("Visible"=TRUE) -> ()  [unwired: 2 in, 2 out]
        n1304 = case shown="\"Multiple\"" "Single/Multiple" {
          frame "Single ", Default {
            n1305 = property on="Single - Graph" class="Ring (strict)"("Visible"=TRUE) -> ()  [unwired: 2 in, 2 out]
            n1306 = local write "Main Tab Display"(T4."Dashboard 3" ("Main Tab Display")) -> ()
          }
          frame "Multiple" {
            n1307 = property on="Single - Graph" class="Ring (strict)"("Visible"=FALSE) -> ()  [unwired: 2 in, 2 out]
            n1308 = local write "Main Tab Display"(T4."Dashboard 2" ("Main Tab Display")) -> ()
          }
        }
      }
    }
    n1309 = local read "Stroke"() -> (w1333:bool)
    n1310 = local read "USERNAME"() -> (w1338:string)
    n1311 = case shown="True" w1336 {
      selector: w1336 -> [_ w1620]
      frame False {
      }
      frame True {
        n1312 = Not(x=w1620) -> (.not. x?=w1619:bool)
        n1313 = local write "Coefficient Of Friction"(w1619) -> ()
        n1314 = local write "Tab Control 2"(T6."Coefficient Of Friction" ("Tab Control 2")) -> ()
      }
    }
    n1315 = case shown="True" w1335 {
      selector: w1335 -> [_ w1617]
      frame False {
      }
      frame True {
        n1316 = Not(x=w1617) -> (.not. x?=w1615:bool)
        n1317 = local write "Air Temperature"(w1615) -> ()
        n1318 = local write "Tab Control 2"(T6."Air Temperature" ("Tab Control 2")) -> ()
      }
    }
    n1319 = case shown="True" w1333 {
      selector: w1333 -> [_ w1611]
      frame False {
      }
      frame True {
        n1320 = Not(x=w1611) -> (.not. x?=w1609:bool)
        n1321 = local write "Stroke"(w1609) -> ()
        n1322 = local write "Tab Control 2"(T6."Stroke" ("Tab Control 2")) -> ()
      }
    }
    n1323 = local write "tested by"(w1338) -> ()
    n1324 = case shown="True" w1334 {
      selector: w1334 -> [_ w1614]
      frame False {
      }
      frame True {
        n1325 = Not(x=w1614) -> (.not. x?=w1612:bool)
        n1326 = local write "Humidity"(w1612) -> ()
        n1327 = local write "Tab Control 2"(T6."Humidity" ("Tab Control 2")) -> ()
      }
    }
    n1328 = case shown="\"Calibration\"" "Main Dashboard Buttons" {
      tunnel: [T2."HOME" ("Main Tab") T2."Test Setup" ("Main Tab") T2."Acquire" ("Main Tab") T2."Adv Scar" ("Main Tab") T2."Adv Scar Report" ("Main Tab") T2."Compare Files" ("Main Tab") T2."Calibration" ("Main Tab") T2."About" ("Main Tab") T2."Advance" ("Main Tab")] -> w1317
      frame "Home", Default {
      }
      frame "Test Setup" {
      }
      frame "Dashboard" {
      }
      frame "Imaging" {
      }
      frame "Report" {
      }
      frame "Analysis" {
      }
      frame "Calibration" {
      }
      frame "About" {
      }
      frame "Advance" {
      }
    }
    n1329 = Wait (ms)(milliseconds to wait=u32 100) -> ()  [unwired: 1 out]
    n1330 = local read "Main Tab Display"() -> (w1337:T4)
    n1331 = local write "Main Tab"(w1317) -> ()
    n1332 = case shown="\"Dashboard 3\"" w1337 {
      frame "Dashboard 1", Default {
        n1333 = property on="Reset Graph" class="Bool (strict)"("Visible"=FALSE) -> ()  [unwired: 2 in, 2 out]
      }
      frame "Dashboard 2" {
        n1334 = property on="Reset Graph" class="Bool (strict)"("Visible"=TRUE) -> ()  [unwired: 2 in, 2 out]
      }
      frame "Dashboard 3" {
        n1335 = property on="Reset Graph" class="Bool (strict)"("Visible"=TRUE) -> ()  [unwired: 2 in, 2 out]
      }
    }
    n1336 = local read "SCAR MEASURMENT"() -> (w1325:enum32{"Auto Scar", "Manual Scar"})
    n1337 = local read "Humidity"() -> (w1339:bool)
    n1338 = local read "Cap Live Image"() -> (w1322:bool)
    n1339 = local read "Sample Temperature"() -> (w1332:bool)
    n1340 = local read "Air Temp vs Humidity"() -> (w1330:bool)
    n1341 = local read "Frequency"() -> (w1331:bool)
    n1342 = case shown="True" w1339 {
      frame False {
        n1343 = local write "Humidity On Command"(TRUE ("Humidity On Command")) -> ()
        n1344 = case shown="True" "Humidity Off Command" {
          selector: "Humidity Off Command" -> [_ w1627]
          frame False {
          }
          frame True {
            n1345 = stacked-sequence {
              frame #0 {
                n1346 = local read "WriteHumidity"() -> (w1629:string[])
                n1347 = Insert Into Array(array=w1629, new element="R;1" ("new element/subarray")) -> (w1628:string[])  [unwired: 1 in]
                n1348 = local write "WriteHumidity"(w1628) -> ()
              }
              frame #1 {
                n1349 = Wait (ms)(milliseconds to wait=u32 2000) -> ()  [unwired: 1 out]
              }
              frame #2 {
                n1350 = local read "WriteHumidity"() -> (w1632:string[])
                n1351 = local read "EVENT LOG"() -> (w1636:string)
                n1352 = call "Event Log.vi"("Content"="Humidity Control Off" ("string"), "EVENT LOG"=w1636) -> ("EVENT LOG"=w1637:string)  [unwired: 8 in, 1 out]
                n1353 = local write "EVENT LOG"(w1637) -> ()
                n1354 = Insert Into Array(array=w1632, new element="R;1" ("new element/subarray")) -> (w1633:string[])  [unwired: 1 in]
                n1355 = local write "WriteHumidity"(w1633) -> ()
              }
            }
            n1356 = Not(x=w1627) -> (.not. x?=w1626:bool)
            n1357 = local write "Humidity Off Command"(w1626) -> ()
          }
        }
      }
      frame True {
        n1358 = local write "Humidity Off Command"(TRUE ("Humidity Off Command")) -> ()
        n1359 = case shown="True" "Humidity On Command" {
          selector: "Humidity On Command" -> [_ w1641]
          frame False {
          }
          frame True {
            n1360 = stacked-sequence {
              frame #0 {
                n1361 = local read "Set Rh"() -> (w1647:dbl)
                n1362 = local read "WriteHumidity"() -> (w1643:string[])
                n1363 = Number To Fractional String(number=w1647, precision (6)=i16 2) -> (F-format string=w1648:string)  [unwired: 2 in]
                n1364 = Concatenate Strings("M;" ("new element/subarray"), w1648) -> (w1646:string)
                n1365 = Insert Into Array(array=w1643, new element=w1646) -> (w1642:string[])  [unwired: 1 in]
                n1366 = local write "WriteHumidity"(w1642) -> ()
              }
              frame #1 {
                n1367 = Wait (ms)(milliseconds to wait=u32 2000) -> ()  [unwired: 1 out]
              }
              frame #2 {
                n1368 = local read "WriteHumidity"() -> (w1651:string[])
                n1369 = local read "Set Rh"() -> (w1655:dbl)
                n1370 = Number To Fractional String(number=w1655, precision (6)=i16 2) -> (F-format string=w1656:string)  [unwired: 2 in]
                n1371 = Concatenate Strings("M;" ("new element/subarray"), w1656) -> (w1654:string)
                n1372 = Insert Into Array(array=w1651, new element=w1654) -> (w1650:string[])  [unwired: 1 in]
                n1373 = local write "WriteHumidity"(w1650) -> ()
              }
              frame #3 {
                n1374 = Wait (ms)(milliseconds to wait=u32 1500) -> ()  [unwired: 1 out]
              }
              frame #4 {
                (unwired) "% RH" ("string")
                (unwired) i16 2 ("precision (6)")
                (unwired) "M;" ("new element/subarray")
                n1375 = local read "Set Rh"() -> (w1665:dbl)
                n1376 = local read "WriteHumidity"() -> (w1658:string[])
                n1377 = Number To Fractional String(number=w1665, precision (6)=i16 2) -> (F-format string=w1662:string)  [unwired: 2 in]
                n1378 = Concatenate Strings("M;" ("new element/subarray"), w1662) -> (w1666:string)
                n1379 = Concatenate Strings("Humidity Set to : " ("string"), w1662, "% RH" ("string")) -> (w1660:string)
                n1380 = Insert Into Array(array=w1658, new element=w1666) -> (w1659:string[])  [unwired: 1 in]
                n1381 = disable-structure shown="Enabled" {
                  frame Enabled {
                    n1382 = local read "EVENT LOG"() -> (w1669:string)
                    n1383 = call "Event Log.vi"("Content"="Humidity Control On", "EVENT LOG"=w1669) -> ("EVENT LOG"=w1670:string)  [unwired: 8 in, 1 out]
                    n1384 = local write "EVENT LOG"(w1670) -> ()
                  }
                  frame Disabled {
                  }
                }
                n1385 = disable-structure shown="Enabled" {
                  disable-tunnel: w1660 -> [_ _]
                  frame Enabled {
                    n1386 = local read "EVENT LOG"() -> (w1672:string)
                    n1387 = call "Event Log.vi"("Content"="Humidity Control On", "EVENT LOG"=w1672) -> ("EVENT LOG"=w1673:string)  [unwired: 8 in, 1 out]
                    n1388 = local write "EVENT LOG"(w1673) -> ()
                  }
                  frame Disabled {
                  }
                }
                n1389 = local write "WriteHumidity"(w1659) -> ()
              }
            }
            n1390 = Not(x=w1641) -> (.not. x?=w1640:bool)
            n1391 = local write "Humidity On Command"(w1640) -> ()
          }
        }
      }
    }
    n1392 = Equal?(x=w1325, y=enum32{"Auto Scar", "Manual Scar"}."Auto Scar" ("SCAR MEASURMENT")) -> (x = y?=w1321:bool)
    n1393 = local read "TEST STANDARD"() -> (w1328:T3)
    n1394 = And(x=w1322, y=w1321) -> (x .and. y?=w1323:bool)
    n1395 = case shown="True" w1323 {
      selector: w1323 -> [_ w1426]
      tunnel: errorcluster {"status"=FALSE, "code"=0, "source"=""} ("error in (no error) 3") -> [_ w1427]
      frame False {
      }
      frame True {
        n1396 = stacked-sequence {
          tunnel: w1427 -> [_ _ _ _ _ _ _ w1475]
          tunnel: w1426 -> [_ _ _ _ _ w1456 _ _]
          frame #0 {
            n1397 = call "CAMERA LIVE FEED FGV.vi"("Enum - Menu"=CAMERA_LIVE_FEED_ENUM."CAMERA MINIMIZE") -> ()  [unwired: 9 in, 2 out]
          }
          frame #1 {
            n1398 = property on="Auto Scar Check  2" class="Clust (strict)"("Visible"=TRUE) -> ()  [unwired: 2 in, 2 out]
          }
          frame #2 {
            n1399 = String To Path(string="C:\\LAB-IQ\\Image Calibrate v01.dcf") -> (path=w1432:path)
            n1400 = Open/Create/Replace File ("Open File")(file path (use dialog)=w1432) -> (refnum out=w1433:refnum<file>)  [unwired: 5 in, 2 out]
            n1401 = for {
              N: 4 -> [_]
              tunnel: w1433 -> [w1439]
              i -> [w1435]
              n1402 = Read from Text File ("Read File")(file (use dialog)=w1439) -> (text=w1440:string)  [unwired: 3 in, 3 out]
              n1403 = String Subset(string=w1440, offset (0)=6, length (rest)=10 ("length (rest)")) -> (substring=w1436:string)
              n1404 = Fract/Exp String To Number(string=w1436) -> (number=w1434:dbl)  [unwired: 3 in, 1 out]
              n1405 = case shown="0" w1435 {
                tunnel: w1434 -> [w1441 w1442 _ w1443 _]
                frame 0 {
                  "5x Gain" <- w1441
                }
                frame 1 {
                  "10x Gain" <- w1442
                }
                frame 2 {
                }
                frame 3 {
                  "100x gain" <- w1443
                }
                frame 4, Default {
                }
              }
            }
          }
          frame #3 {
            n1406 = local read "FILE 3"() -> (w1449:string)
            n1407 = call <vilib>:"Trim Whitespace.vi"("string"="C:\\LAB-IQ\\images\\") -> ("trimmed string"=w1451:string)  [unwired: 1 in]
            n1408 = String To Path(string=w1451) -> (path=w1450:path)
            n1409 = Concatenate Strings(w1449, ".png" ("string")) -> (w1448:string)
            n1410 = Build Path(base path=w1450, name or relative path=w1448) -> (appended path=w1446:path)
            "Image path" <- w1446
            n1411 = Path To String(path=w1446) -> (string=w1445:string)
            n1412 = call "CAMERA LIVE FEED FGV.vi"("Enum - Menu"=CAMERA_LIVE_FEED_ENUM."CAMERA SAVE", "Image Path"=w1445) -> ()  [unwired: 8 in, 2 out]
          }
          frame #4 {
            n1413 = One Button Dialog(message="Image saved successfully") -> ()  [unwired: 1 in, 1 out]
          }
          frame #5 {
            n1414 = local read "TEST STANDARD"() -> (w1455:T3)
            n1415 = local read "Magnification len live scar"() -> (w1467:string)
            n1416 = Not(x=w1456) -> (.not. x?=w1457:bool)
            n1417 = local write "Cap Live Image"(w1457) -> ()
            n1418 = case shown="\"ISO 12156\"" w1455 {
              tunnel: ["ASTM D6079" "ISO 12156"] -> w1454
              frame "ASTM D6079", Default {
              }
              frame "ISO 12156" {
              }
            }
            n1419 = case shown="\"5x\", Default" w1467 {
              tunnel: [w1470 w1471] -> w1466
              frame "5x", Default {
                n1420 = local read "5x Gain"() -> (w1470:dbl)
              }
              frame "10x" {
                # "5x"
                n1421 = local read "10x Gain"() -> (w1471:dbl)
              }
            }
            n1422 = local read "Image path"() -> (w1465:path)
            n1423 = local read "FILE 3"() -> (w1458:string)
            n1424 = call "EDGE DETCTION.vi"("GAIN VALUE"=w1466, "Image Path"=w1465) -> ("error out"=w1464:errorcluster, "return value"=w1463:cluster{string, string, dbl, dbl, dbl})  [unwired: 8 in]
            n1425 = Bundle By Name(cluster=T27 {"File Name"="", "Test Method"="", "Operator"="", "Fuel Description"="", "Date and time"=""} ("Main Ref"), "File Name"=w1458, "Test Method"=w1454) -> (w1459:T27)
            n1426 = call "duf file read.vi"("error in (no error)"=w1464, "Main Ref"=w1459) -> ("error out"=w1462:errorcluster, "Main Ref 2"=w1460:T27)  [unwired: 8 in]
            n1427 = call "EDGE DETECTION REPORT.vi"("error in (no error)"=w1462, "return value 2"=w1463, "Main Ref"=w1460) -> ()  [unwired: 8 in, 1 out]
          }
          frame #6 {
            n1428 = property on="Auto Scar Check  2" class="Clust (strict)"("Visible"=FALSE) -> ()  [unwired: 2 in, 2 out]
          }
          frame #7 {
            n1429 = call "CAMERA LIVE FEED FGV.vi"("Enum - Menu"=CAMERA_LIVE_FEED_ENUM."CAMERA MINIMIZE", "error in (no error)"=w1475) -> ()  [unwired: 8 in, 2 out]
            n1430 = local write "Main Dashboard Buttons"(T1."Home" ("Main Dashboard Buttons")) -> ()
            n1431 = local write "Main Tab"(T2."HOME" ("Main Tab")) -> ()
          }
        }
      }
    }
    n1432 = local read "Heater Button"() -> (w1329:bool)
    n1433 = case shown="True" w1331 {
      selector: w1331 -> [_ w1605]
      frame False {
      }
      frame True {
        n1434 = Not(x=w1605) -> (.not. x?=w1603:bool)
        n1435 = local write "Frequency"(w1603) -> ()
        n1436 = local write "Tab Control 2"(T6."Frequency" ("Tab Control 2")) -> ()
      }
    }
    n1437 = case shown="True" w1330 {
      selector: w1330 -> [_ w1602]
      frame False {
      }
      frame True {
        n1438 = Not(x=w1602) -> (.not. x?=w1600:bool)
        n1439 = local write "Air Temp vs Humidity"(w1600) -> ()
        n1440 = local write "Tab Control 2"(T6."Air Temp vs Rh" ("Tab Control 2")) -> ()
      }
    }
    n1441 = case shown="True" w1332 {
      selector: w1332 -> [_ w1608]
      frame False {
      }
      frame True {
        n1442 = Not(x=w1608) -> (.not. x?=w1606:bool)
        n1443 = local write "Sample Temperature"(w1606) -> ()
        n1444 = local write "Tab Control 2"(T6."Sample Temperature" ("Tab Control 2")) -> ()
      }
    }
    n1445 = case shown="\"Custom\"" w1328 {
      frame "ASTM D6079", Default {
        w1581 = "ASTM D6079 TEST CONDITIONS" ("Standard 2")
        n1446 = local write "Standard 2"(w1581) -> ()
        n1447 = local write "Standard"(w1581) -> ()
      }
      frame "ISO 12156" {
        w1582 = "ISO 12156 TEST CONDITIONS" ("Standard 2")
        n1448 = local write "Standard 2"(w1582) -> ()
        n1449 = local write "Standard"(w1582) -> ()
      }
      frame "CEC F-096-A-06" {
        w1583 = "CEC F-096-A-06 TEST CONDITIONS" ("Standard 2")
        n1450 = local write "Standard 2"(w1583) -> ()
        n1451 = local write "Standard"(w1583) -> ()
      }
      frame "Custom" {
        w1584 = "CUSTOM TEST CONDITIONS" ("Standard 2")
        n1452 = local write "Standard 2"(w1584) -> ()
        n1453 = local write "Standard"(w1584) -> ()
      }
    }
    n1454 = case shown="True" w1329 {
      frame False {
        n1455 = local write "Temperature On Command"(TRUE ("Temperature On Command")) -> ()
        n1456 = case shown="True" "Temperature Off Command" {
          selector: "Temperature Off Command" -> [_ w1588]
          frame False {
          }
          frame True {
            n1457 = Not(x=w1588) -> (.not. x?=w1587:bool)
            n1458 = local read "EVENT LOG"() -> (w1591:string)
            n1459 = local write "Temperature Off Command"(w1587) -> ()
            n1460 = call "Event Log.vi"("Content"="Heater Off", "EVENT LOG"=w1591) -> ("EVENT LOG"=w1590:string)  [unwired: 8 in, 1 out]
            n1461 = local write "EVENT LOG"(w1590) -> ()
          }
        }
      }
      frame True {
        n1462 = local write "Temperature Off Command"(TRUE ("Temperature Off Command")) -> ()
        n1463 = case shown="True" "Temperature On Command" {
          selector: "Temperature On Command" -> [_ w1595]
          frame False {
          }
          frame True {
            n1464 = Not(x=w1595) -> (.not. x?=w1594:bool)
            n1465 = local write "Temperature On Command"(w1594) -> ()
            n1466 = disable-structure shown="Enabled" {
              disable-tunnel: "Heater On" -> [w1597 _]
              frame Enabled {
                n1467 = local read "EVENT LOG"() -> (w1598:string)
                n1468 = call "Event Log.vi"("Content"=w1597, "EVENT LOG"=w1598) -> ("EVENT LOG"=w1599:string)  [unwired: 8 in, 1 out]
                n1469 = local write "EVENT LOG"(w1599) -> ()
              }
              frame Disabled {
              }
            }
          }
        }
      }
    }
    n1470 = local read "Main Tab"() -> (w1320:T2)
    n1471 = case shown="\"About\"" w1320 {
      frame "HOME", Default {
        w1362 = T19."Enabled" ("Disabled")
        n1472 = local read "Service Password enable"() -> (w1364:bool)
        n1473 = property on="Imaging" class="Bool (strict)"("DisabledEnum"=w1362) -> ()  [unwired: 2 in, 2 out]
        n1474 = property on="Dashboard" class="Bool (strict)"("DisabledEnum"=w1362) -> ()  [unwired: 2 in, 2 out]
        n1475 = property on="Test Setup" class="Bool (strict)"("DisabledEnum"=w1362) -> ()  [unwired: 2 in, 2 out]
        n1476 = property on="Analysis" class="Bool (strict)"("DisabledEnum"=w1362) -> ()  [unwired: 2 in, 2 out]
        n1477 = property on="Home" class="Bool (strict)"("DisabledEnum"=w1362) -> ()  [unwired: 2 in, 2 out]
        n1478 = property on="Report" class="Bool (strict)"("DisabledEnum"=w1362) -> ()  [unwired: 2 in, 2 out]
        n1479 = property on="Main Dashboard Buttons" class="RadioBtnsControl (strict)"("DisabledEnum"=w1362) -> ()  [unwired: 2 in, 2 out]
        n1480 = property on="Calibration" class="Bool (strict)"("DisabledEnum"=w1362) -> ()  [unwired: 2 in, 2 out]
        n1481 = case shown="True" w1364 {
